vi "SeCrTS-DD NS Receiver.vi"(8 "error in":errorcluster) -> (0 "error out":errorcluster)   [LabVIEW 2022 SP3]
uses:
  Globals/SeCrTS-DD globals.vi
  <resource>/objmgr/ni.dex.rc
panel:
  out "timed out?":bool
  out "x":u32
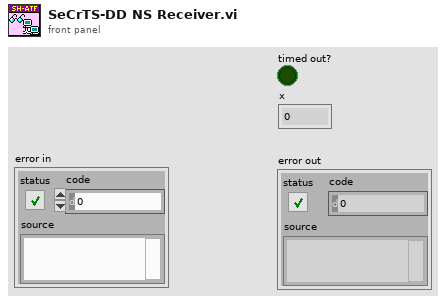
[diagram p1: front panel]
types:
  T1 = cluster{"In Progress":bool, "reader url":refnum<k21>}
  T2 = enum16{"Initialize", "Wait for connection", "Send data", "Exit", "Receive Data"}
  T3 = typedef "SeCrTS-Notifier Ref.ctl" = cluster{"DO NOT S":refnum<notifier>, "AI V NOT P":refnum<notifier>, "AI C NOT S":refnum<notifier>, "TC NOT P":refnum<notifier>, "DI NOT S":refnum<notifier>, "DI NOT P":refnum<notifier>, "DO NOT P":refnum<notifier>, "AI C NOT  P":refnum<notifier>}
  T4 = cluster{"AI_V_Data":waveform(dbl)[][], "AI_C_Data":waveform(dbl)[][], "AO_Data":waveform(dbl)[][], "DO_Data":waveform(dbl)[][], "DI_Data":digitalwaveform[][], "ACC_Data":waveform(dbl)[][], "TC Data":waveform(dbl)[][], "Drive_A_C":waveform(dbl)[][], "Drive_A_D":waveform(dbl)[][], "Drive_L_C":waveform(dbl)[][], "Drive_L_D":waveform(dbl)[][], "RT Time":timestamp}
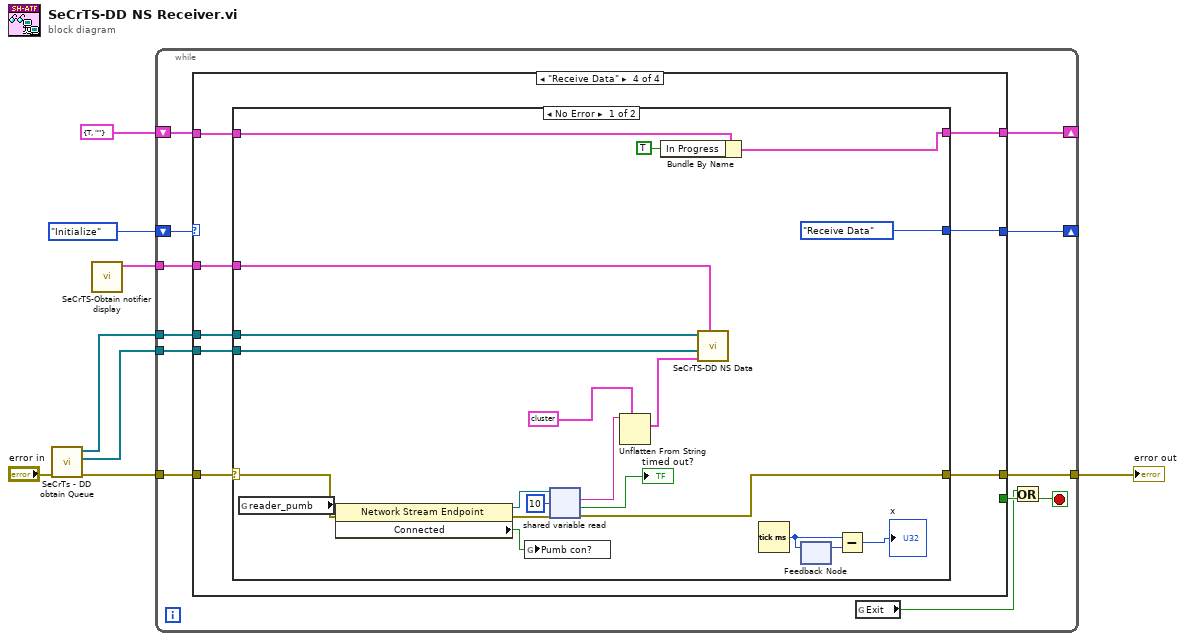
[diagram p0: block diagram]
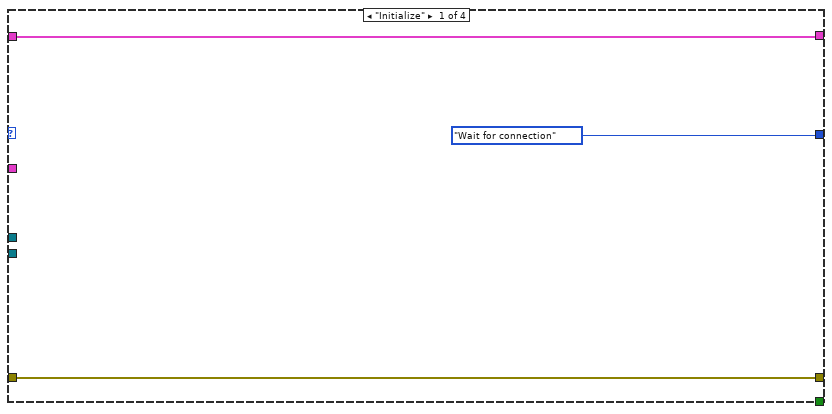
[diagram p2: hidden frame]
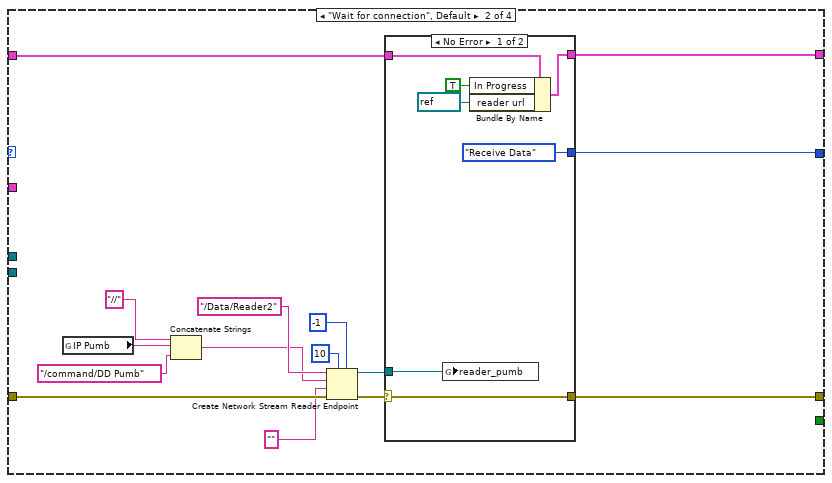
[diagram p3: hidden frame]
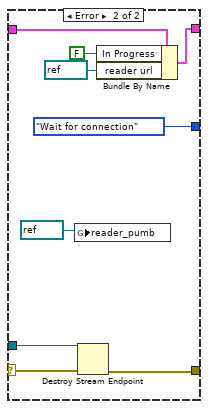
[diagram p4: hidden frame]
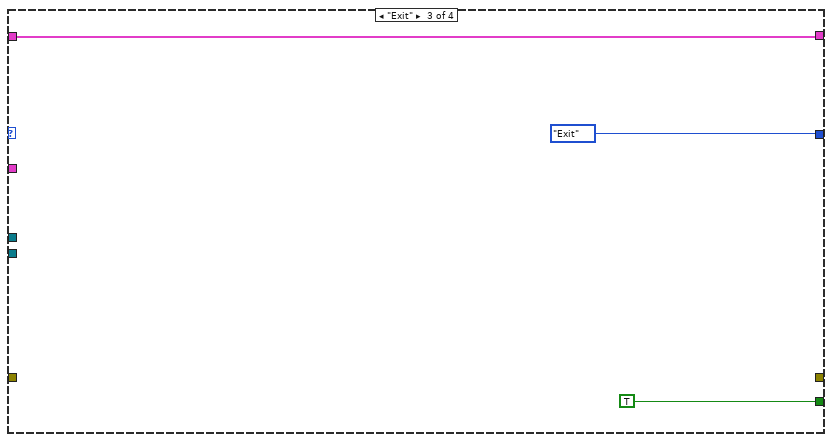
[diagram p5: hidden frame]
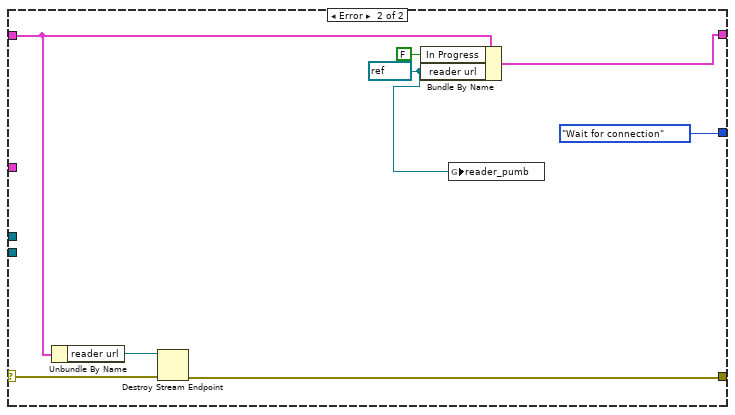
[diagram p6: hidden frame]
diagram:
  n1 = call "SeCrTs - DD obtain Queue.vi"("error in"="error in") -> ("error out"=w4:errorcluster, "AI_V_Data P\nAI_C_Data P\nAO_Data P\nDO_Data P\nACC_Data P\nTC Data P\nDrive_A_C \nDrive_A_D\nAI_C_Data S\nDO_Data S"=w1:refnum<queue>[], "DI P\nDI S"=w2:refnum<queue>[])  [unwired: 8 in]
  n2 = call "SeCrTS-Obtain notifier display.vi"() -> ("NOT DIS Out"=w5:T3)  [unwired: 11 in]
  n3 = while {
    shift-right: [w18] -> _
    shift-left: T2."Initialize" -> [w20]
    shift-right: [w16] -> _
    shift-left: T1 {"In Progress"=TRUE, "reader url"=""} -> [w17]
    tunnel: w4 -> [w15]
    tunnel: [w14] -> w6
    tunnel: w5 -> [w11]
    tunnel: w2 -> [w10]
    tunnel: w1 -> [w9]
    stop <- w13 stop-if-true
    n4 = case shown="\"Receive Data\"" w20 {
      tunnel: [_ _ TRUE _] -> w19
      tunnel: [T2."Wait for connection" w34 T2."Exit" w62] -> w18
      tunnel: w17 -> [w23 w38 w56 w65]
      tunnel: [w23 w37 w56 w63] -> w16
      tunnel: w15 -> [w21 w36 _ w64]
      tunnel: [w21 w35 _ w61] -> w14
      tunnel: w11 -> [_ _ _ w60]
      tunnel: w10 -> [_ _ _ w59]
      tunnel: w9 -> [_ _ _ w58]
      frame "Initialize" {
      }
      frame "Wait for connection", Default {
        n5 = global read "SeCrTS-DD globals.vi" "IP Pumb"() -> (w25:string)
        n6 = Concatenate Strings("//" ("string"), w25, "/command/DD Pumb" ("reader url")) -> (w27:string)
        n7 = Create Network Stream Reader Endpoint(5:-1 ("timeout in ms (-1)"), 7:10 ("reader buffer size"), 8:w36, 9:"", 10:w27, 11:"/Data/Reader2" ("writer name")) -> (0:w31:errorcluster, 3:w32:refnum<k21>)  [unwired: 1 in]
        n8 = case shown="No Error" w31 {
          selector: w31 -> [w42 w50]
          tunnel: w38 -> [w45 w54]
          tunnel: w32 -> [w40 w51]
          tunnel: [w43 w53] -> w37
          tunnel: [w42 w49] -> w35
          tunnel: [T2."Receive Data" T2."Wait for connection"] -> w34
          frame No Error {
            n9 = global write "SeCrTS-DD globals.vi" "reader_pumb"(w40) -> ()
            n10 = Bundle By Name(cluster=w45, "In Progress"=TRUE, "reader url"=refnum<k21> refnum) -> (w43:T1)
          }
          frame Error {
            n11 = global write "SeCrTS-DD globals.vi" "reader_pumb"(refnum<k21> refnum ("reader")) -> ()
            n12 = Destroy Stream Endpoint(8:w50, 11:w51) -> (0:w49:errorcluster)
            n13 = Bundle By Name(cluster=w54, "In Progress"=FALSE, "reader url"=refnum<k21> refnum) -> (w53:T1)
          }
        }
      }
      frame "Exit" {
      }
      frame "Receive Data" {
        n14 = case shown="No Error" w64 {
          selector: w64 -> [w81 w89]
          tunnel: w65 -> [w86 w92]
          tunnel: [w85 w94] -> w63
          tunnel: [T2."Receive Data" T2."Wait for connection"] -> w62
          tunnel: [w78 w88] -> w61
          tunnel: w60 -> [w70 _]
          tunnel: w59 -> [w69 _]
          tunnel: w58 -> [w68 _]
          frame No Error {
            n15 = global read "SeCrTS-DD globals.vi" "reader_pumb"() -> (w79:refnum<k21>)
            n16 = property class="Network Stream Endpoint"(reference=w79, error in=w81) -> (reference out=w83:refnum<k21>, error out=w80:errorcluster, "Connected"=w77:bool)
            n17 = global write "SeCrTS-DD globals.vi" "Pumb con?"(w77) -> ()
            n18 = shared-variable-read(w83, w80, 10 ("timeout ms (-1)")) -> (w78:errorcluster, →"timed out?":bool, w73:string)  [unwired: 1 out]
            n19 = Unflatten From String(type=T4 data[101864B] ("data out"), binary string=w73) -> (value=w66:T4)  [unwired: 3 in, 2 out]
            n20 = Bundle By Name(cluster=w86, "In Progress"=TRUE) -> (w85:T1)
            n21 = call "SeCrTS-DD NS Data.vi"("NOT DIS Out"=w70, "value"=w66, "AI_V_Data P\nAI_C_Data P\nAO_Data P\nDO_Data P\nACC_Data P\nTC Data P\nDrive_A_C \nDrive_A_D\nAI_C_Data S\nDO_Data S"=w68, "DI P\nDI S"=w69) -> ()  [unwired: 8 in]
            n22 = Tick Count (ms)() -> (millisecond timer value=w75:u32)
            n23 = feedback-in #1(w75) -> ()
            n24 = feedback #1() -> (w76:u32)  [unwired: 1 in]
            n25 = Subtract(x=w75, y=w76) -> (x-y=→"x":u32)
          }
          frame Error {
            w87 = refnum<k21> refnum ("reader url")
            n26 = Unbundle By Name(w92) -> ("reader url"=w91:refnum<k21>)
            n27 = Destroy Stream Endpoint(8:w89, 11:w91) -> (0:w88:errorcluster)
            n28 = Bundle By Name(cluster=w92, "In Progress"=FALSE, "reader url"=w87) -> (w94:T1)
            n29 = global write "SeCrTS-DD globals.vi" "reader_pumb"(w87) -> ()
          }
        }
      }
    }
    n30 = global read "SeCrTS-DD globals.vi" "Exit"() -> (w12:bool)
    n31 = Or(x=w12, y=w19) -> (x .or. y?=w13:bool)
  }
  "error out" <- w6
